vi "CreateDetector.vi"(6 "Detector Settings":T1={"Refine Edges (Default: True)"=TRUE, "Threads (Default: 1)"=1, "Decimate (Default: 1)"=1.0, "Blur (Default: 0)"=0.0, "Bits (Default: 2)"=2} {"Threads (Default: 1)" min=1}, 8 "error in (no error)":errorcluster, 11 "Family":T2) -> (0 "error out":errorcluster, 3 "Apriltag Detector":refnum<class "AprilTag Detector.lvclass">)   [LabVIEW 2020, in "feature_detection.lvlib" / "AprilTag Detector.lvclass"]
uses:
  AprilTag Detector.lvclass
  AprilTag Families.ctl
  Detector Settings.ctl
  AprilTag Detector.lvclass/AprilTag Detector.ctl
  common/common.lvlib
  common/bin/gartoolkit_fd_32-1.dll
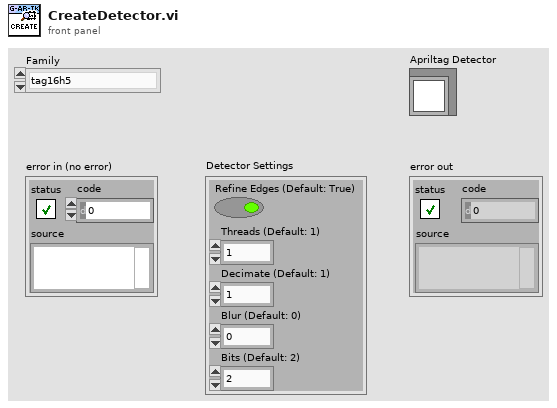
[diagram p1: front panel]
types:
  T1 = typedef "feature_detection.lvlib/AprilTag Detector.lvclass/Detector Settings.ctl" = cluster{"Refine Edges (Default: True)":bool, "Threads (Default: 1)":u8, "Decimate (Default: 1)":sgl, "Blur (Default: 0)":sgl, "Bits (Default: 2)":u8}
  T2 = typedef "feature_detection.lvlib/AprilTag Detector.lvclass/AprilTag Families.ctl" = enum8{"tag16h5", "tag25h9", "tag36h11", "tagCircle21h7", "tagCircle49h12", "tagCustom48h12", "tagStandard41h12", "tagStandard52h13"}
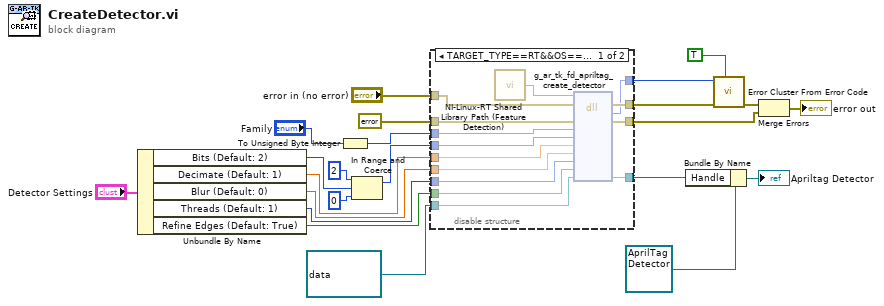
[diagram p0: block diagram]
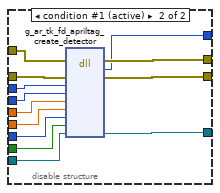
[diagram p2: hidden frame]
diagram:
  n1 = Unbundle By Name("Detector Settings") -> ("Bits (Default: 2)"=w17:u8, "Decimate (Default: 1)"=w10:sgl, "Blur (Default: 0)"=w9:sgl, "Threads (Default: 1)"=w8:u8, "Refine Edges (Default: True)"=w7:bool)
  n2 = To Unsigned Byte Integer(number="Family") -> (unsigned 8bit integer=w12:u8)
  n3 = In Range and Coerce(upper limit=u8 2, x=w17, lower limit=u8 0) -> (coerced(x)=w11:u8)  [unwired: 1 out]
  n4 = disable-structure shown="TARGET_TYPE==RT&&OS==Linux" {
    disable-tunnel: "error in (no error)" -> [w36 w50]
    disable-tunnel: errorcluster {"status"=FALSE, "code"=0, "source"=""} ("error constant") -> [w35 w49]
    disable-tunnel: w12 -> [w34 w48]
    disable-tunnel: w11 -> [w33 w47]
    disable-tunnel: w10 -> [w32 w46]
    disable-tunnel: w9 -> [w31 w45]
    disable-tunnel: w8 -> [w30 w44]
    disable-tunnel: w7 -> [w29 w43]
    disable-tunnel: refnum<data-value> refnum ("EDVR") -> [w28 w42]
    disable-tunnel: [w27 w41] -> w5
    disable-tunnel: [w26 w40] -> w4
    disable-tunnel: [w25 w39] -> w3
    disable-tunnel: [w24 w38] -> w2
    frame condition #0 {
      n5 = call "NI-Linux-RT Shared Library Path (Feature Detection).vi"() -> ("Path"=w37:path)
      n6 = dll-call lib="?" fn="g_ar_tk_fd_apriltag_create_detector" ("g_ar_toolkit.*.*:g_ar_tk_capture_context_create")(path in=w37, error in=w36, "error_cluster"=w35, "tag_family"=w34, "bits"=w33, "decimate"=w32, "blur"=w31, "threads"=w30, "refine_edges"=w29, "EDVR"=w28) -> (error out=w27:errorcluster, w26:i32, "error_cluster"=w25:errorcluster, "EDVR"=w24:refnum<data-value>)  [unwired: 7 in, 1 out]
    }
    frame condition #1 (active) {
      n7 = dll-call lib="C:/serenial/lib/g-augmented-reality-toolkit/LabVIEW/common/bin/gartoolkit_fd_*-1.*" fn="g_ar_tk_fd_apriltag_create_detector" ("g_ar_toolkit.*.*:g_ar_tk_capture_context_create")(error in=w50, "error_cluster"=w49, "tag_family"=w48, "bits"=w47, "decimate"=w46, "blur"=w45, "threads"=w44, "refine_edges"=w43, "EDVR"=w42) -> (error out=w41:errorcluster, w40:i32, "error_cluster"=w39:errorcluster, "EDVR"=w38:refnum<data-value>)  [unwired: 8 in, 1 out]
    }
  }
  n8 = Bundle By Name(cluster=refnum<class "AprilTag Detector.lvclass"> refnum ("CameraManager out"), "Handle"=w2) -> (→"Apriltag Detector":refnum<class "AprilTag Detector.lvclass">)
  n9 = call <vilib>:"Error Cluster From Error Code.vi"("show call chain? (False)"=TRUE, "error in (no error)"=w5, "error code (0)"=w4) -> ("error out"=w22:errorcluster)  [unwired: 6 in]
  n10 = Merge Errors(w22, w3) -> (→"error out":errorcluster)
